vi "uService GUI.vi"(8 "error in (no error)":errorcluster, 11 "uService Template in":refnum<class "Kasli Server.lvclass">=refnum) -> (3 "uService Template out":refnum<class "Kasli Server.lvclass">)   [LabVIEW 2020, in "CIRCUS_uServices.lvlib" / "Kasli Server.lvlib" / "Kasli Server.lvclass"]
uses:
  Kasli Server.lvclass
  TALOS/TALOS_PPL.lvlibp/Father of all uServices/Father of all uServices/Father of all uServices.lvclass
  C:/Users/marco/Documents/GitHub_Lab/CIRCUS/TALOS/TALOS_PPL.lvlibp/Ancestor/Ancestor/Ancestor.lvclass
  C:/Users/marco/Documents/GitHub_Lab/CIRCUS/TALOS/Actor Framework.lvlibp/1abvi3w/vi.lib/ActorFramework/Actor/Actor.lvclass
  C:/Users/marco/Documents/GitHub_Lab/CIRCUS/TALOS/TALOS_PPL.lvlibp/Father of all uServices/Father of all uServices/Father of all uServices.lvclass
panel:
  in  "Message":string
  in  "Kasli Name":string
  in  "Send":bool
  out "Safe Mode":bool
  in  "Stop":bool
  out "uService ID":string
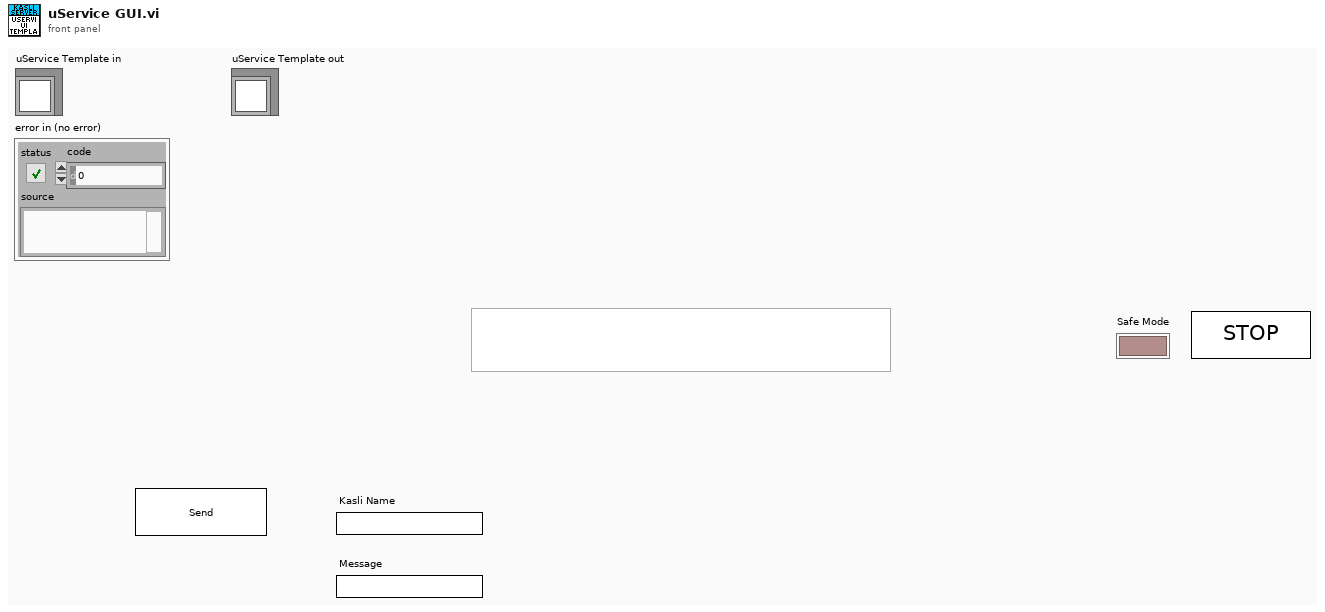
[diagram p1: front panel]
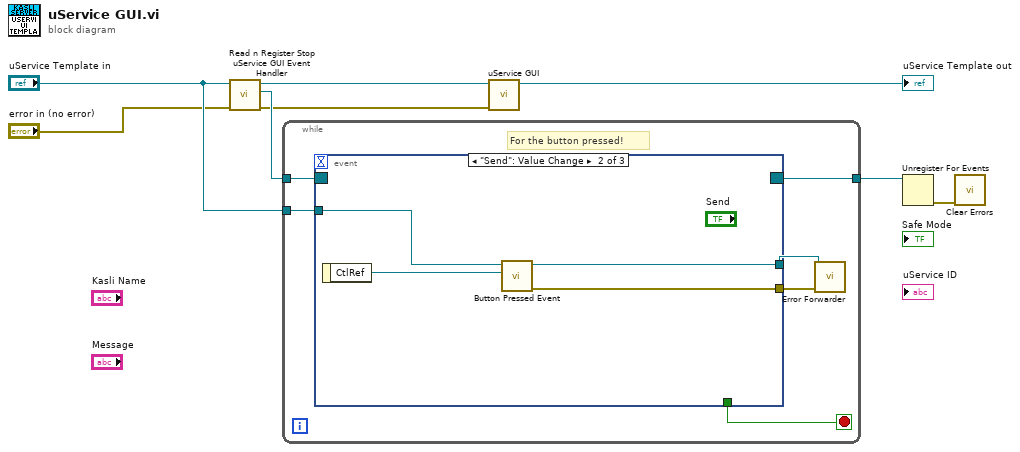
[diagram p0: block diagram]
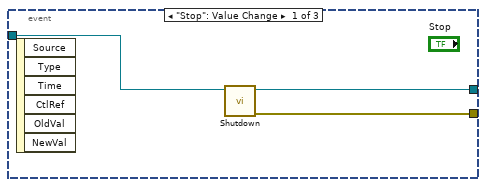
[diagram p2: hidden frame]
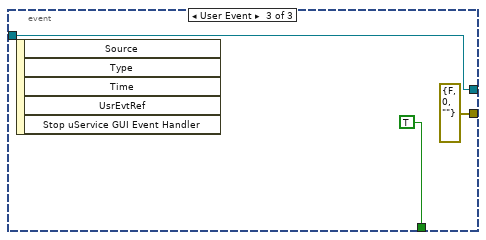
[diagram p3: hidden frame]
diagram:
  n1 = call-dynamic "Read n Register Stop uService GUI Event Handler .vi"("error in (no error)"="error in (no error)", "uService Template in"="uService Template in") -> ("error out"=w2:errorcluster, "Stop uService GUI Event Ref"=w6:refnum<event-registration>, "uService Template out"=w4:refnum<class "Kasli Server.lvclass">)  [unwired: 7 in]
  n2 = while {
    tunnel: [w14] -> w7
    tunnel: "uService Template in" -> [w12]
    tunnel: w6 -> [w11]
    stop <- w13 stop-if-true
    # "For the button pressed!"
    n3 = event shown="[1] \"Send\": Value Change" {
      selector: w11 -> [_ _ _]
      dyn-events: [_ _ _] -> w14
      timeout: _ -> [_ _ _]
      tunnel: w12 -> [w17 w21 w23]
      tunnel: [_ _ TRUE] -> w13
      tunnel: [w16 w19 w23] -> w10
      tunnel: [w15 w18 errorcluster {"status"=FALSE, "code"=0, "source"=""} ("error out")] -> w9
      event "Stop": Value Change {
        n4 = event-data() -> ()  [unwired: 1 in, 6 out]
        n5 = call "Shutdown.vi"("Father of all uServices in"=w17) -> ("error out"=w15:errorcluster, "Father of all uServices out"=w16:refnum<class "Father of all uServices.lvclass">)  [unwired: 9 in]
      }
      event "Send": Value Change {
        n6 = event-data() -> ("CtlRef"=w20:refnum<vi>)  [unwired: 1 in]
        n7 = call-dynamic "Button Pressed Event.vi"("CtlRef"=w20, "uService Template in"=w21) -> ("error out"=w18:errorcluster, "uService Template out"=w19:refnum<class "Kasli Server.lvclass">)  [unwired: 8 in]
      }
      event User Event {
        n8 = event-data() -> ()  [unwired: 1 in, 5 out]
      }
    }
    n9 = call "Error Forwarder.vi"("error in (no error)"=w9, "Father of all uServices in"=w10) -> ()  [unwired: 10 in]
  }
  n10 = call-parent "uService GUI.vi"("error in (no error)"=w2, "uService Template in"=w4) -> ("uService Template out"=→"uService Template out":refnum<class "Kasli Server.lvclass">)  [unwired: 9 in]
  n11 = Unregister For Events(event registration refnum=w7) -> (error out=w1:errorcluster)  [unwired: 1 in]
  n12 = call <vilib>:"Clear Errors.vi"("error in (no error)"=w1) -> ()  [unwired: 5 in, 2 out]
